vi "Read Waveform In Fast Mode.vi"(5 "Number Of Points (64)":u32=64, 7 "Data Sample Rate (0: 62.5 mHz)":u16(ring) items=["62.5 mHz", "125 mHz", "250 mHz", "500 mHz", "1 Hz", "2 Hz", "4 Hz", "8 Hz", "16 Hz", "32 Hz", "64 Hz", "128 Hz", "256 Hz", "512 Hz", "Trigger"], 8 "Error In (no error)":errorcluster, 9 "Second Output Mode (3: Y)":u16(ring)=3 items=["R [V]", "Theta", "X", "Y"], 10 "First Output Mode (2: X)":u16(ring)=2 items=["R [V]", "Theta", "X", "Y"], 11 "VISA Resource Name":refnum<visa-resource-name>) -> (0 "Error Out":errorcluster, 1 "Second Output Mode Array":dbl[](array[numeric]) format="%.2p", 2 "First Output Mode Array":dbl[](array[numeric]) format="%.2p", 3 "VISA Resource Name Out":refnum<visa-resource-name>)   [LabVIEW 2010, in "Stanford Research 844.lvlib"]
doc: "This VI starts measurement in fast mode and reads the points, which are sent in this mode from instrument.\n\nNote: Timeout needed for this operation is set automatically. (it could take few minutes to complete the operation e.g. time for operation in seconds = number of points / data sample rate in hertz)\n\nImportant: This VI is for GPIB only."
uses:
  <instrlib>/Stanford Research 844/Stanford Research 844.lvlib
panel:
  # "GPIB only !!!"
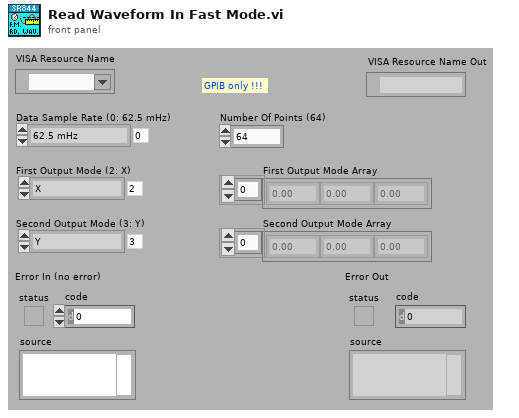
[diagram p1: front panel]
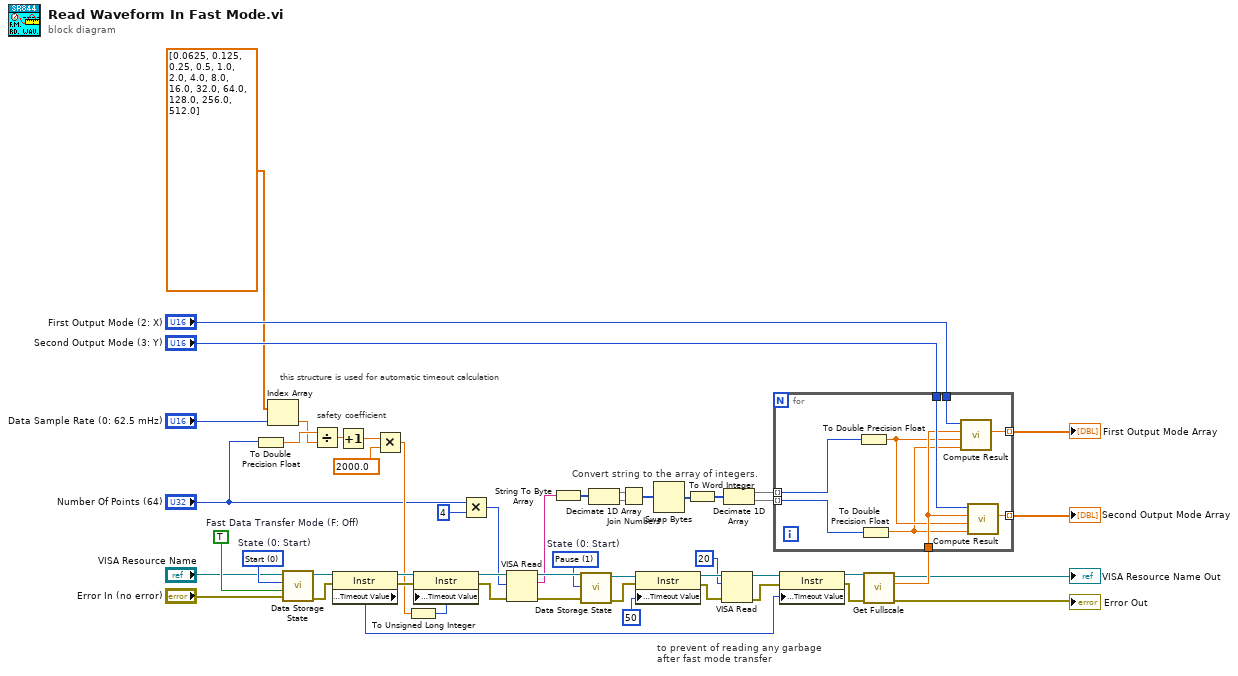
[diagram p0: block diagram]
diagram:
  w34 = u16 0 items=["Start", "Pause", "Reset"]  # State (0: Start)
  w31 = u16 1 items=["Start", "Pause", "Reset"]  # State (0: Start)
  w52 = TRUE  # Fast Data Transfer Mode (F: Off)
  # "to prevent of reading any garbage \nafter fast mode transfer"
  # "safety coefficient"
  # "this structure is used for automatic timeout calculation"
  # "Convert string to the array of integers."
  n1 = To Double Precision Float(number="Number Of Points (64)") -> (double precision float=w3:dbl)
  n2 = Index Array(array=dbl[] [0.0625, 0.125, 0.25, 0.5, 1.0, 2.0, 4.0, 8.0, 16.0, 32.0, 64.0, 128.0, 256.0, 512.0], index="Data Sample Rate (0: 62.5 mHz)") -> (element=w2:dbl)
  n3 = call <instrlib>:"Data Storage State.vi"("Error In (no error)"="Error In (no error)", "Fast Data Transfer Mode (F: Off)"=w52, "State (0: Start)"=w34, "VISA Resource Name"="VISA Resource Name") -> ("Error Out"=w50:errorcluster, "VISA Resource Name Out"=w51:refnum<visa-resource-name>)  [unwired: 6 in]
  n4 = Divide(x=w3, y=w2) -> (x/y=w4:dbl)
  n5 = property class="Instr"(reference=w51, error in=w50) -> (reference out=w49:refnum<visa-resource-name>, error out=w48:errorcluster, "General Settings:Timeout Value"=w38:u32)
  n6 = Increment(x=w4) -> (x+1=w17:dbl)
  n7 = Multiply(x=w17, y=2000.0) -> (x*y=w16:dbl)
  n8 = To Unsigned Long Integer(number=w16) -> (unsigned 32bit integer=w37:u32)
  n9 = property class="Instr"(reference=w49, error in=w48, "General Settings:Timeout Value"=w37) -> (reference out=w47:refnum<visa-resource-name>, error out=w46:errorcluster)
  n10 = Multiply(x="Number Of Points (64)", y=u32 4) -> (x*y=w23:u32)
  n11 = VISA Read(VISA resource name=w47, byte count=w23, error in (no error)=w46) -> (VISA resource name out=w45:refnum<visa-resource-name>, read buffer=w41:string, error out=w44:errorcluster)  [unwired: 1 out]
  n12 = String To Byte Array(string=w41) -> (unsigned byte array=w39:u8[])
  n13 = call <instrlib>:"Data Storage State.vi"("Error In (no error)"=w44, "State (0: Start)"=w31, "VISA Resource Name"=w45) -> ("Error Out"=w11:errorcluster, "VISA Resource Name Out"=w10:refnum<visa-resource-name>)  [unwired: 7 in]
  n14 = Decimate 1D Array(w39) -> (w33:u8[], w32:u8[])
  n15 = Join Numbers(hi=w33, lo=w32) -> ((hi.lo)=w30:u16[])
  n16 = property class="Instr"(reference=w10, error in=w11, "General Settings:Timeout Value"=u32 50) -> (reference out=w13:refnum<visa-resource-name>, error out=w8:errorcluster)
  n17 = Swap Bytes(anything=w30) -> (byte swapped=w29:u16[])
  n18 = To Word Integer(number=w29) -> (16bit integer=w15:i16[])
  n19 = VISA Read(VISA resource name=w13, byte count=u32 20 ("byte count (0)"), error in (no error)=w8) -> (VISA resource name out=w9:refnum<visa-resource-name>, error out=w1:errorcluster)  [unwired: 2 out]
  n20 = Decimate 1D Array(w15) -> (w40:i16[], w36:i16[])
  n21 = property class="Instr"(reference=w9, error in=w1, "General Settings:Timeout Value"=w38) -> (reference out=w43:refnum<visa-resource-name>, error out=w42:errorcluster)
  n22 = call <instrlib>:"Get Fullscale.vi"("Error In (no error)"=w42, "VISA Resource Name"=w43) -> ("Error Out"=→"Error Out":errorcluster, "Full Scale"=w35:dbl, "VISA Resource Name Out"=→"VISA Resource Name Out":refnum<visa-resource-name>)  [unwired: 7 in]
  n23 = for {
    tunnel: w40 -> [w61] mode=indexing
    tunnel: w36 -> [w60] mode=indexing
    tunnel: w35 -> [w55]
    tunnel: [w57] -> w21 mode=indexing
    tunnel: [w59] -> w22 mode=indexing
    tunnel: "First Output Mode (2: X)" -> [w58]
    tunnel: "Second Output Mode (3: Y)" -> [w56]
    n24 = To Double Precision Float(number=w61) -> (double precision float=w54:dbl)
    n25 = To Double Precision Float(number=w60) -> (double precision float=w53:dbl)
    n26 = call <instrlib>:"Compute Result.vi"("Y"=w53, "X"=w54, "Full Scale"=w55, "Mode (2: X)"=w58) -> ("Computed Value"=w59:dbl)  [unwired: 7 in]
    n27 = call <instrlib>:"Compute Result.vi"("Y"=w53, "X"=w54, "Full Scale"=w55, "Mode (2: X)"=w56) -> ("Computed Value"=w57:dbl)  [unwired: 7 in]
  }
  "First Output Mode Array" <- w22
  "Second Output Mode Array" <- w21
